vi "CS-4 Set Units.vi"(3 "error in (no error)":errorcluster, 4 "units":enum16{"Amps", "Kilogauss", "Tesla"}(ring)=enum."Kilogauss", 5 "VISA session":refnum<visa-resource-name>) -> (0 "error out":errorcluster, 2 "dup VISA session":refnum<visa-resource-name>)   [LabVIEW 2016]
doc: "CS-4 Set Units.vi selects Amps, kiloGauss or Tesla for all input and display operations."
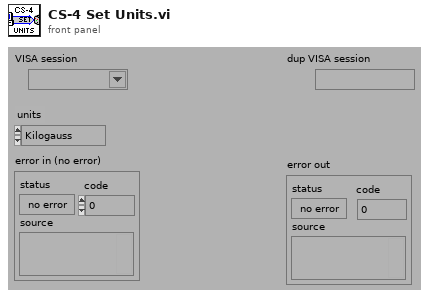
[diagram p1: front panel]
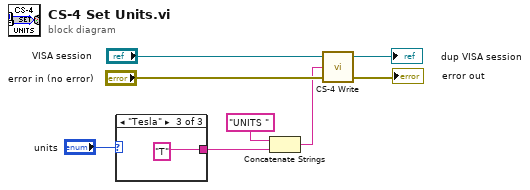
[diagram p0: block diagram]
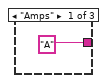
[diagram p2: hidden frame]
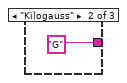
[diagram p3: hidden frame]
diagram:
  n1 = case shown="\"Tesla\"" "units" {
    tunnel: ["A" "G" "T"] -> w2
    frame "Amps" {
    }
    frame "Kilogauss" {
    }
    frame "Tesla" {
    }
  }
  n2 = Concatenate Strings("UNITS ", w2) -> (w6:string)
  n3 = call "CS-4 Write.vi"("error in (no error)"="error in (no error)", "write buffer (\"\")"=w6, "VISA session"="VISA session") -> ("error out"=→"error out":errorcluster, "dup VISA session"=→"dup VISA session":refnum<visa-resource-name>)  [unwired: 1 out]
